vi "Initialise State.vi"(8 "Input (use dialog)":path=path "C:/Users/craig.walker/Documents/GitHub/lv2019-Advent-of-Code-2021/23/input.txt", 9 "Sample":string, 10 "Sample?":bool, 11 "Part 1?":bool) -> (3 "State":cluster{"Hallway":string[], "Rooms":string[][]})   [LabVIEW 2019, in "23.lvlib"]
uses:
  23.lvlib
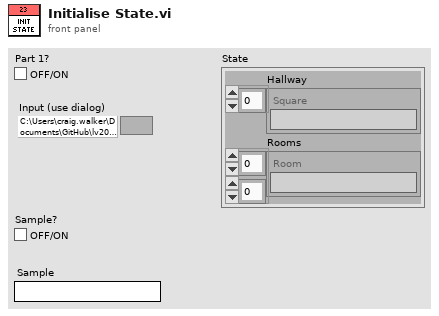
[diagram p1: front panel]
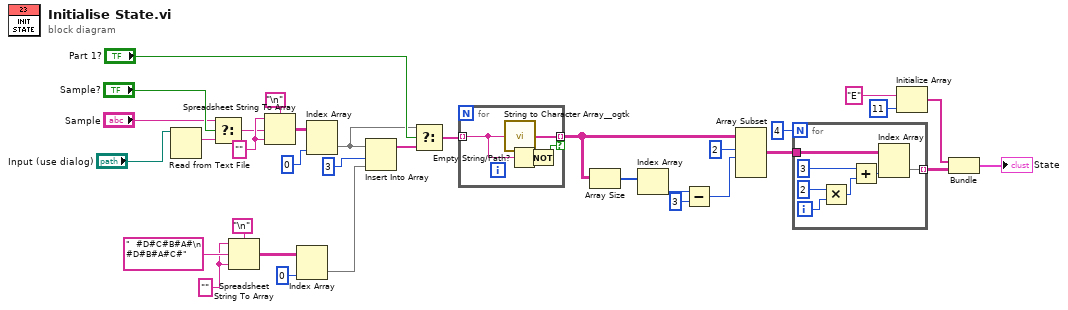
[diagram p0: block diagram]
diagram:
  w11 = "" ("format string")
  w6 = "" ("format string")
  n1 = Read from Text File(file (use dialog)="Input (use dialog)") -> (text=w2:string)  [unwired: 3 in, 3 out]
  n2 = Select(t="Sample", s="Sample?", f=w2) -> (s? t:f=w5:string)
  n3 = Spreadsheet String To Array(delimiter (Tab)="\n", format string=w11, spreadsheet string="  #D#C#B#A#\n  #D#B#A#C#", array type (2D Dbl)=w11) -> (array=w15:string[][])
  n4 = Spreadsheet String To Array(delimiter (Tab)="\n", format string=w6, spreadsheet string=w5, array type (2D Dbl)=w6) -> (array=w8:string[][])
  n5 = Index Array(array=w15, index (col)=0 ("disabled index (col)")) -> (element=w16:string[])  [unwired: 1 in]
  n6 = Index Array(array=w8, index (col)=0 ("disabled index (col)")) -> (element=w20:string[])  [unwired: 1 in]
  n7 = Insert Into Array(array=w20, index=3, new element=w16) -> (w19:string[])
  n8 = Select(t=w20, s="Part 1?", f=w19) -> (s? t:f=w18:string[])
  n9 = for {
    tunnel: w18 -> [w36] mode=indexing
    tunnel: [w37] -> w22 mode=indexing if=w34
    n10 = call <userlib>:"String to Character Array__ogtk.vi"("Input String"=w36) -> ("Character Array"=w37:string[])
    n11 = Empty String/Path?(string/path=w36) -> (empty?=w35:bool)
    n12 = Not(x=w35) -> (.not. x?=w34:bool)
  }
  n13 = Array Size(array=w22) -> (size(s)=w23:i32[])
  n14 = Index Array(array=w23) -> (element=w26:i32)  [unwired: 1 in]
  n15 = Subtract(x=w26, y=3) -> (x-y=w27:i32)
  n16 = Array Subset(array=w22, index (row)=2, length (row)=w27) -> (w25:string[][])  [unwired: 2 in]
  n17 = for {
    N: 4 -> [_]
    tunnel: w25 -> [w44]
    tunnel: [w38] -> w30 mode=indexing
    i -> [w41]
    n18 = Multiply(x=2, y=w41) -> (x*y=w39:i32)
    n19 = Add(x=3 ("disabled index (col)"), y=w39) -> (x+y=w42:i32)
    n20 = Index Array(array=w44, index (col)=w42) -> (element=w38:string[])  [unwired: 1 in]
  }
  n21 = Initialize Array("E", 11 ("dimension size")) -> (w31:string[])
  n22 = Bundle(w31, w30) -> (→"State":cluster{string[], string[][]})  [unwired: 1 in]
